vi "Associated Research 78XX Series Run Test and Collect Data.vi"(8 "error in (no error)":errorcluster, 11 "VISA resource name":refnum<visa-resource-name>) -> (0 "error out":errorcluster)   [LabVIEW 2020]
doc: "This VI is an example to start a TEST, check the status of the test, and record data after a test. It is required that \"Saving and Creating a file\" is run before this."
uses:
  <instrlib>/Associated Research 78XX Series/Public/Configure/Steps/Low Level/ULTRA Test Type.ctl
  <instrlib>/Associated Research 78XX Series/Associated Research 78XX Series.lvlib
panel:
  out "File Name":string
  out "Test Data Status?":T2
  out "Read all Buffer":T3(array[cluster])
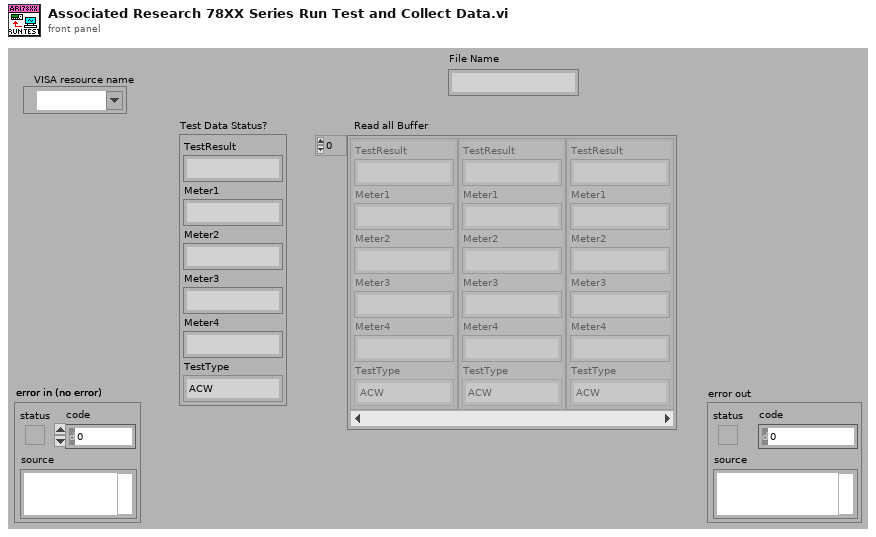
[diagram p1: front panel]
types:
  T1 = typedef "Associated Research 78XX Series.lvlib/ULTRA Test Type.ctl" = enum16{"ACW", "CONT", "DCW", "-DCW", "IR"}
  T2 = cluster{"TestResult":string, "Meter1":string, "Meter2":string, "Meter3":string, "Meter4":string, "TestType":T1}
  T3 = cluster{"TestResult":string, "Meter1":string, "Meter2":string, "Meter3":string, "Meter4":string, "TestType":T1}[]
  T4 = cluster{"All Pass":bool, "Fail":bool, "Abort":bool, "Test in Process":bool, "Message Available":bool, "Event Summary Bit":bool, "Not Used":bool, "Prompt":bool}
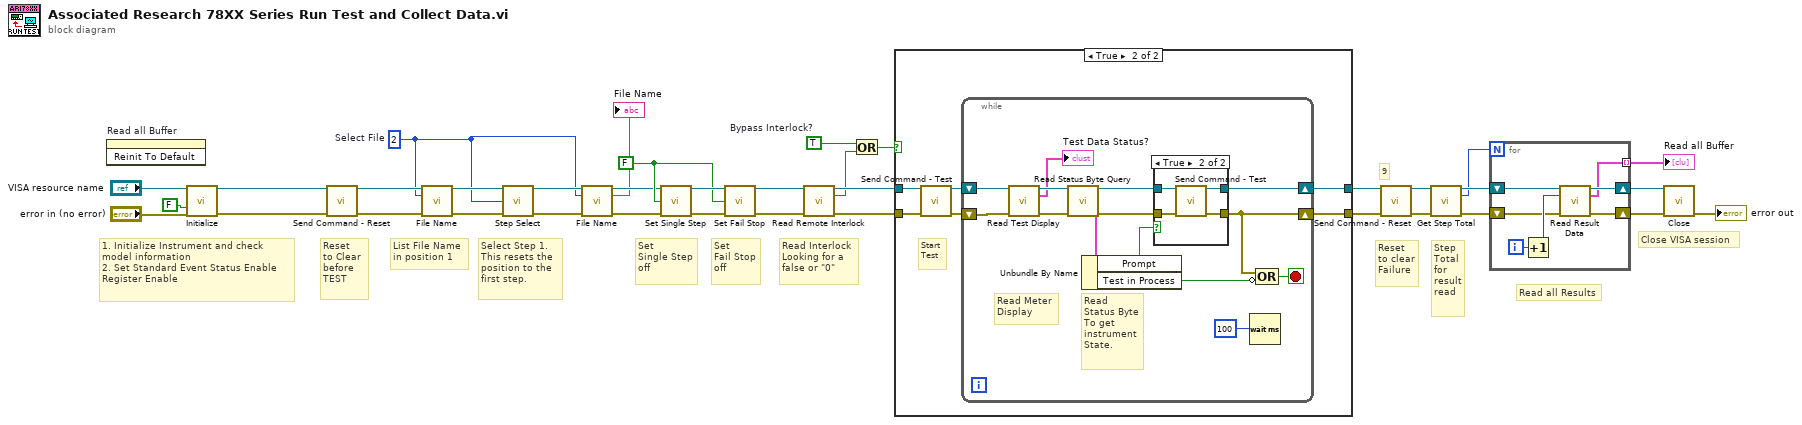
[diagram p0: block diagram]
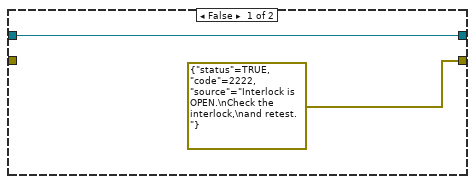
[diagram p2: hidden frame]
diagram:
  w8 = TRUE  # Bypass Interlock?
  w13 = FALSE ("Single Step On/OFF (F:Off)")
  w2 = 2  # Select File
  # "Close VISA session"
  # "Read all Results"
  # "Step\nTotal\nfor \nresult\nread"
  # "Reset\nto clear\nFailure"
  # "Read Interlock\nLooking for a\nfalse or \"0\""
  # "Set\nFail Stop\noff"
  # "Set \nSingle Step\noff"
  # "Select Step 1.\nThis resets the\nposition to the \nfirst step."
  # "List File Name\nin position 1"
  # "Reset\nto Clear \nbefore \nTEST"
  # "1. Initialize Instrument and check model information\n2. Set Standard Event Status Enable Register Enable"
  # "9"
  n1 = invoke on="Read all Buffer" class="Arr (strict)" method="Reinit To Default"() -> ()  [unwired: 3 in, 3 out]
  n2 = call <instrlib>:"Initialize.vi"("VISA resource name"="VISA resource name", "Reset (True)"=FALSE, "error in (no error)"="error in (no error)") -> ("VISA resource name out"=w7:refnum<visa-resource-name>, "error out"=w6:errorcluster)  [unwired: 10 in, 1 out]
  n3 = call <instrlib>:"Send Command - Reset.vi"("VISA resource name"=w7, "error in (no error)"=w6) -> ("VISA resource name out"=w15:refnum<visa-resource-name>, "error out"=w14:errorcluster)  [unwired: 12 in]
  n4 = call <instrlib>:"File Name.vi"("VISA resource name"=w15, "File Number"=w2, "error in (no error)"=w14) -> ("VISA resource name out"=w24:refnum<visa-resource-name>, "error out"=w23:errorcluster)  [unwired: 10 in, 1 out]
  n5 = call <instrlib>:"Step Select.vi"("VISA resource name"=w24, "Step Number (1)"=w2, "error in (no error)"=w23) -> ("VISA resource name out"=w4:refnum<visa-resource-name>, "error out"=w22:errorcluster)  [unwired: 11 in]
  n6 = call <instrlib>:"File Name.vi"("VISA resource name"=w4, "File Number"=w2, "error in (no error)"=w22) -> ("VISA resource name out"=w3:refnum<visa-resource-name>, "File Name"=→"File Name":string, "error out"=w5:errorcluster)  [unwired: 10 in]
  n7 = call <instrlib>:"Set Single Step.vi"("VISA resource name"=w3, "Single Step On/OFF (F:Off)"=w13, "error in (no error)"=w5) -> ("VISA resource name out"=w21:refnum<visa-resource-name>, "error out"=w20:errorcluster)  [unwired: 11 in]
  n8 = call <instrlib>:"Set Fail Stop.vi"("VISA resource name"=w21, "Fail Stop On/OFF (F:Off)"=w13, "error in (no error)"=w20) -> ("VISA resource name out"=w18:refnum<visa-resource-name>, "error out"=w19:errorcluster)  [unwired: 11 in]
  n9 = call <instrlib>:"Read Remote Interlock.vi"("VISA resource name"=w18, "error in (no error)"=w19) -> ("VISA resource name out"=w17:refnum<visa-resource-name>, "Remote Interlock"=w12:bool, "error out"=w16:errorcluster)  [unwired: 11 in]
  n10 = Or(x=w8, y=w12) -> (x .or. y?=w9:bool)
  n11 = case shown="True" w9 {
    tunnel: [w38 w43] -> w36
    tunnel: [errorcluster {"status"=TRUE, "code"=2222, "source"="Interlock is OPEN.\nCheck the interlock,\nand retest."} ("error out") w42] -> w35
    tunnel: w17 -> [w38 w41]
    tunnel: w16 -> [_ w40]
    frame False {
    }
    frame True {
      # "Start\nTest"
      n12 = call <instrlib>:"Send Command - Test.vi"("VISA resource name"=w41, "error in (no error)"=w40) -> ("VISA resource name out"=w44:refnum<visa-resource-name>, "error out"=w39:errorcluster)  [unwired: 12 in]
      n13 = while {
        shift-left: w39 -> [w48]
        shift-right: [w53] -> w42
        shift-left: w44 -> [w49]
        shift-right: [w54] -> w43
        stop <- w57 stop-if-true
        # "Read Meter\nDisplay"
        # "Read \nStatus Byte\nTo get \ninstrument\nState."
        n14 = call <instrlib>:"Read Test Display.vi"("VISA resource name"=w49, "error in (no error)"=w48) -> ("VISA resource name out"=w47:refnum<visa-resource-name>, "Test Data Cluster"=→"Test Data Status?":T2, "error out"=w45:errorcluster)  [unwired: 11 in]
        n15 = call <instrlib>:"Read Status Byte Query.vi"("VISA resource name"=w47, "error in (no error)"=w45) -> ("VISA resource name out"=w51:refnum<visa-resource-name>, "Status Byte Register"=w56:T4, "error out"=w50:errorcluster)  [unwired: 11 in]
        n16 = Unbundle By Name(w56) -> ("Prompt"=w52:bool, "Test in Process"=w55:bool)
        n17 = case shown="True" w52 {
          tunnel: w51 -> [w60 w64]
          tunnel: [w60 w63] -> w54
          tunnel: w50 -> [w59 w62]
          tunnel: [w59 w61] -> w53
          frame False {
          }
          frame True {
            n18 = call <instrlib>:"Send Command - Test.vi"("VISA resource name"=w64, "error in (no error)"=w62) -> ("VISA resource name out"=w63:refnum<visa-resource-name>, "error out"=w61:errorcluster)  [unwired: 12 in]
          }
        }
        n19 = Wait (ms)(milliseconds to wait=u32 100) -> ()  [unwired: 1 out]
        n20 = Compound Arithmetic op=OR(w53, invert w55) -> (w57:bool)
      }
    }
  }
  n21 = call <instrlib>:"Send Command - Reset.vi"("VISA resource name"=w36, "error in (no error)"=w35) -> ("VISA resource name out"=w30:refnum<visa-resource-name>, "error out"=w29:errorcluster)  [unwired: 12 in]
  n22 = call <instrlib>:"Get Step Total.vi"("VISA resource name"=w30, "error in (no error)"=w29) -> ("VISA resource name out"=w28:refnum<visa-resource-name>, "# of Steps"=w26:i32, "error out"=w27:errorcluster)  [unwired: 11 in]
  n23 = for {
    N: w26 -> [_]
    shift-right: [w69] -> w11
    shift-left: w28 -> [w70]
    shift-right: [w67] -> w10
    shift-left: w27 -> [w65]
    tunnel: [w68] -> w25 mode=indexing
    i -> [w71]
    n24 = Increment(x=w71) -> (x+1=w66:i32)
    n25 = call <instrlib>:"Read Result Data.vi"("VISA resource name"=w70, "Result Number (1-200) (1)"=w66, "error in (no error)"=w65) -> ("VISA resource name out"=w69:refnum<visa-resource-name>, "Test Data Cluster"=w68:T2, "error out"=w67:errorcluster)  [unwired: 10 in]
  }
  "Read all Buffer" <- w25
  n26 = call <instrlib>:"Close.vi"("VISA resource name"=w11, "error in (no error)"=w10) -> ("error out"=→"error out":errorcluster)  [unwired: 13 in]
